vi "AsciiLookupTable.vi"(12 "Input 0x ascii":string="0x12 0x52 0x41 0x47 0x45 0x5F 0x53 0x59 0x53 0x54 0x45 0x4D 0x53 0x5F 0x38 0x36 0x33 0x57 0x33") -> (6 "result string":string)   [LabVIEW 2018]
panel:
  out "length ( bytes)":u32
  out "Length ( bytes)":string
  out "array":string[](array[string])
  out "after substring":string
  # "Ascii hex to string"
  # "Vi was made to parse data for the UCD 9090 but can be modified for other ascii parsing requirements"
  # "0x12 0x52 0x41 0x47 0x45 0x5F 0x53 0x59 0x53 0x54 0x45 0x4D 0x53 0x5F 0x38 0x36 0x33 0x57 0x33 = RAGE_SYSTEMS_863W3"
  # "0x0A 0x30 0x31 0x39 0x35 0x30 0x5F 0x4E 0x42 0x50 0x54 0x6D 0xFF = 01950_NBPT"
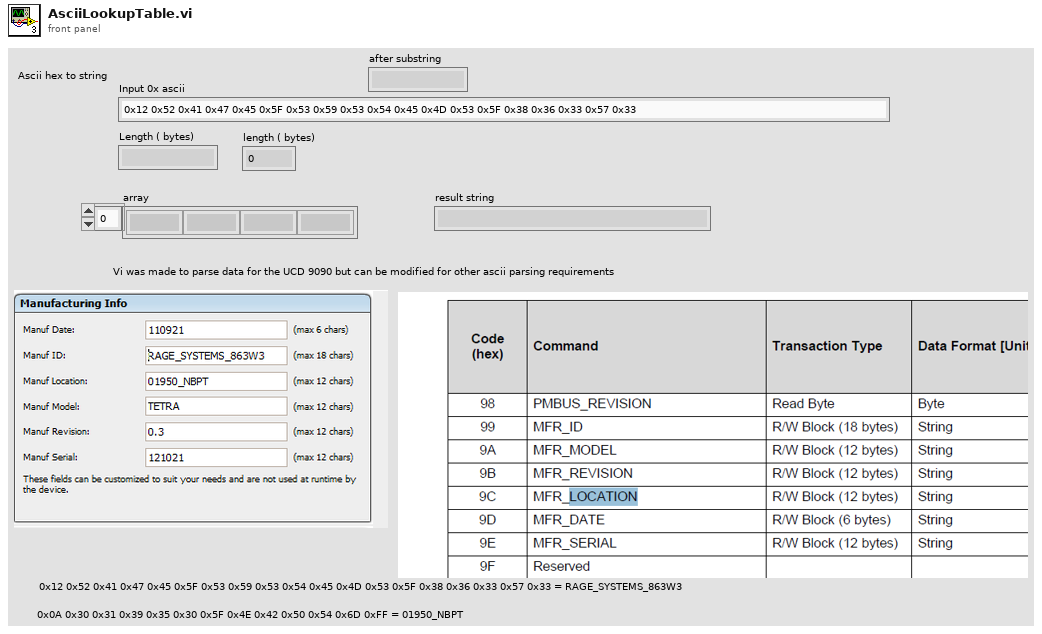
[diagram p1: front panel]
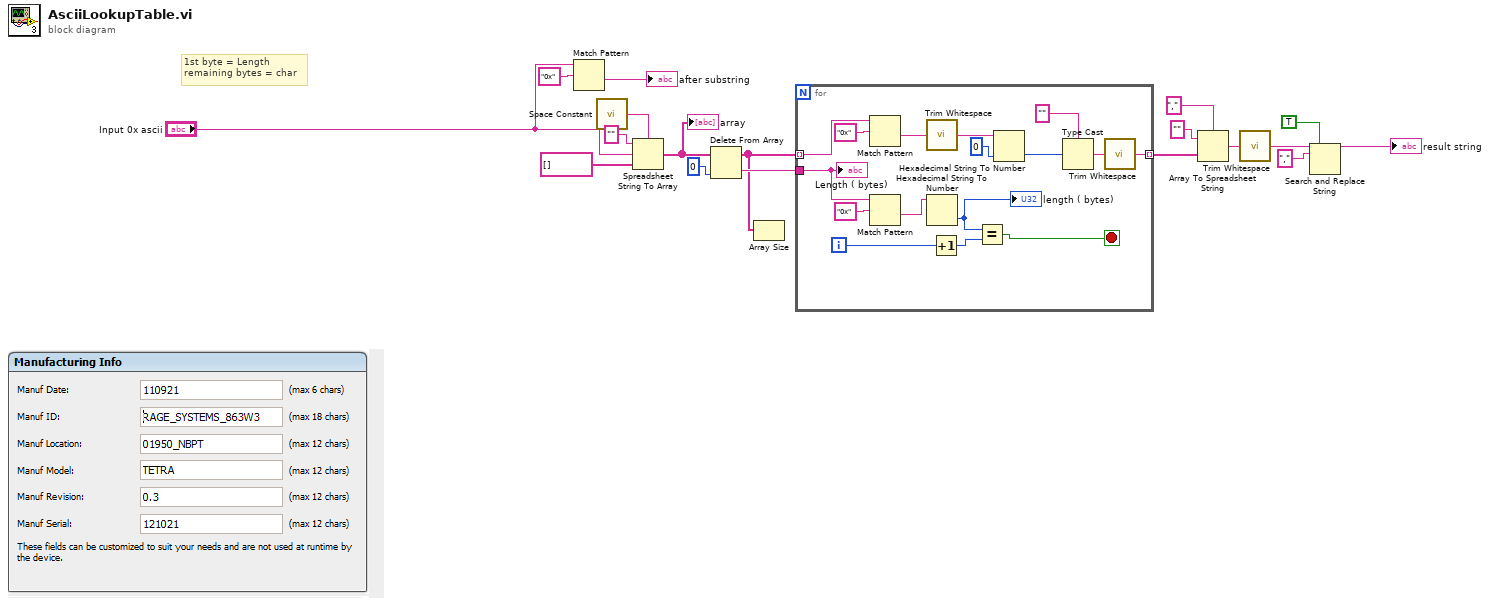
[diagram p0: block diagram]
diagram:
  # "1st byte = Length\nremaining bytes = char"
  n1 = Match Pattern(string="Input 0x ascii", regular expression="0x") -> (after substring=→"after substring":string)  [unwired: 1 in, 3 out]
  n2 = call <vilib>:"Space Constant.vi"() -> ("String"=w13:string)
  n3 = Spreadsheet String To Array(delimiter (Tab)=w13, format string="", spreadsheet string="Input 0x ascii", array type (2D Dbl)=string[] []) -> (array=w12:string[])
  "array" <- w12
  n4 = Delete From Array(array=w12, index=0 ("index (row)")) -> (deleted portion=w2:string, array with subset deleted=w1:string[])  [unwired: 1 in]
  n5 = Array Size(array=w1) -> ()  [unwired: 1 out]
  n6 = for {
    tunnel: w1 -> [w32] mode=indexing
    tunnel: [w27] -> w3 mode=indexing
    tunnel: w2 -> [w24]
    i -> [w22]
    stop <- w20 stop-if-true
    n7 = Match Pattern(string=w32, regular expression="0x") -> (after substring=w29:string)  [unwired: 1 in, 3 out]
    n8 = Match Pattern(string=w24, regular expression="0x") -> (after substring=w23:string)  [unwired: 1 in, 3 out]
    n9 = call <vilib>:"Trim Whitespace.vi"("string"=w29) -> ("trimmed string"=w26:string)  [unwired: 1 in]
    n10 = Hexadecimal String To Number(string=w23) -> (number=w21:u32)  [unwired: 2 in, 1 out]
    "length ( bytes)" <- w21
    n11 = Increment(x=w22) -> (x+1=w19:i32)
    n12 = Equal?(x=w21, y=w19) -> (x = y?=w20:bool)
    n13 = Hexadecimal String To Number(string=w26, default (0uL)=u8 0 ("default (0 U32)")) -> (number=w31:u8)  [unwired: 1 in, 1 out]
    n14 = Type Cast(type="", x=w31) -> (*(type *) &x=w33:string)
    n15 = call <vilib>:"Trim Whitespace.vi"("string"=w33) -> ("trimmed string"=w27:string)  [unwired: 1 in]
    "Length ( bytes)" <- w24
  }
  n16 = Array To Spreadsheet String(delimiter (Tab)=",", array=w3, 3:"" ("format string")) -> (spreadsheet string=w10:string)
  n17 = call <vilib>:"Trim Whitespace.vi"("string"=w10) -> ("trimmed string"=w8:string)  [unwired: 1 in]
  n18 = Search and Replace String(replace all?=TRUE ("replace all? (F)"), input string=w8, search string="," ("replace string (\"\")")) -> (result string=→"result string":string)  [unwired: 5 in, 3 out]
